vi "Event_Update.vi"(6 "CMD":T1(ring)=enum."Update_Event", 8 "Error In":errorcluster, 9 "Update?":bool=TRUE, 10 "Event Ref":refnum<vi>, 11 "Event":string) -> (0 "Error Out":errorcluster)   [LabVIEW 2025]
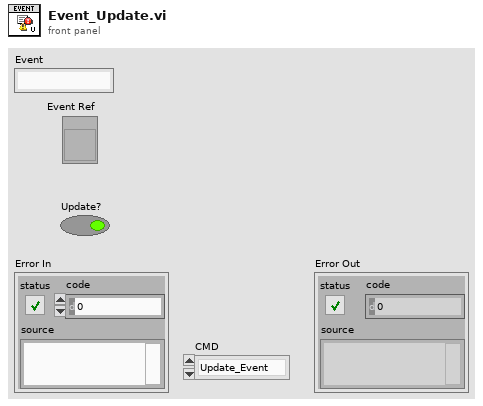
[diagram p1: front panel]
types:
  T1 = enum16{"Init", "Update_Event", "Publish_Event", "Reset"}
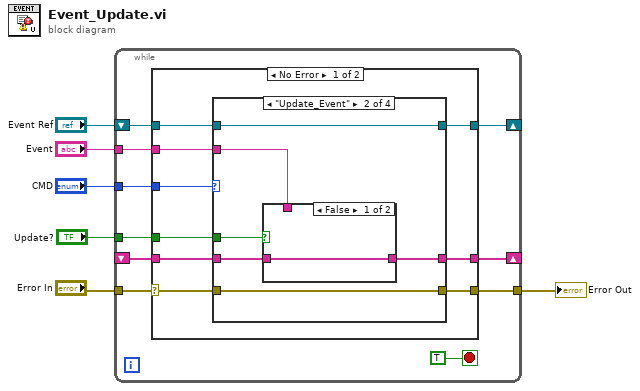
[diagram p0: block diagram]
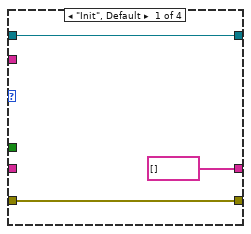
[diagram p2: hidden frame]
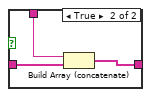
[diagram p3: hidden frame]
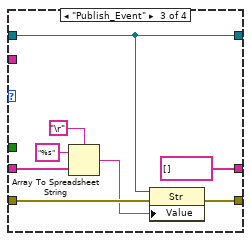
[diagram p4: hidden frame]
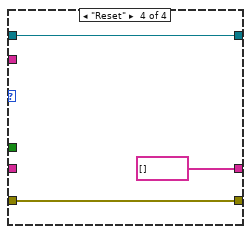
[diagram p5: hidden frame]
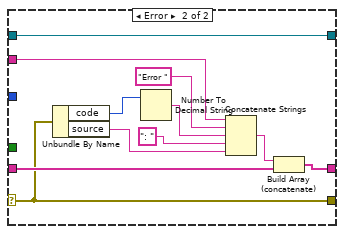
[diagram p6: hidden frame]
diagram:
  n1 = while {
    tunnel: "CMD" -> [w16]
    shift-right: [w14] -> _
    shift-left: _ -> [w12]
    tunnel: "Event" -> [w13]
    tunnel: [w11] -> w3
    tunnel: "Error In" -> [w8]
    shift-right: [w9] -> _
    shift-left: "Event Ref" -> [w10]
    tunnel: "Update?" -> [w7]
    stop <- TRUE stop-if-true
    n2 = case shown="No Error" w8 {
      selector: w8 -> [w18 w59]
      tunnel: w16 -> [w25 _]
      tunnel: [w24 w55] -> w14
      tunnel: w13 -> [w23 w50]
      tunnel: w12 -> [w22 w60]
      tunnel: [w21 w59] -> w11
      tunnel: w10 -> [w20 w51]
      tunnel: [w19 w51] -> w9
      tunnel: w7 -> [w17 _]
      frame No Error {
        n3 = case shown="\"Update_Event\"" w25 {
          tunnel: [string[] [] w34 string[] [] string[] []] -> w24
          tunnel: w23 -> [_ w31 _ _]
          tunnel: w22 -> [_ w30 w42 _]
          tunnel: [w27 w33 w44 w49] -> w21
          tunnel: w18 -> [w27 w33 w45 w49]
          tunnel: w20 -> [w26 w32 w43 w47]
          tunnel: [w26 w32 w43 w47] -> w19
          tunnel: w17 -> [_ w29 _ _]
          frame "Init", Default {
          }
          frame "Update_Event" {
            n4 = case shown="False" w29 {
              tunnel: [w35 w38] -> w34
              tunnel: w31 -> [_ w37]
              tunnel: w30 -> [w35 w36]
              frame False {
              }
              frame True {
                n5 = Build Array (concatenate)(w37, w36) -> (w38:string[])
              }
            }
          }
          frame "Publish_Event" {
            n6 = Array To Spreadsheet String(delimiter (Tab)="\r", array=w42, 3:"%s" ("format string")) -> (spreadsheet string=w40:string)
            n7 = property class="Str"(reference=w43, error in=w45, "Value"=w40) -> (error out=w44:errorcluster)  [unwired: 1 out]
          }
          frame "Reset" {
          }
        }
      }
      frame Error {
        n8 = Unbundle By Name(w59) -> ("code"=w54:i32, "source"=w57:string)
        n9 = Number To Decimal String(number=w54) -> (decimal integer string=w53:string)  [unwired: 1 in]
        n10 = Concatenate Strings(w50, "Error ", w53, ": " ("string"), w57) -> (w58:string)
        n11 = Build Array (concatenate)(w58, w60) -> (w55:string[])
      }
    }
  }
  "Error Out" <- w3
